vi "Get Required Driver Type.vi"(8 "error in (no error)":errorcluster, 11 "Multi Instrument Msg in":refnum<class "Multi Instrument Msg.lvclass">) -> (0 "error out":errorcluster, 2 "Required Driver Type":refnum<class "Instrument Driver.lvclass">, 3 "Multi Instrument Msg out":refnum<class "Multi Instrument Msg.lvclass">)   [LabVIEW 2020, in "Instrument Handler.lvlib" / "Multi Instrument Msg.lvclass"]
doc: "Get the Required Driver Type for execution of the Instrument Msg.\n\nThis implementation does nothing."
uses:
  Multi Instrument Msg.lvclass
  PPL/HDH.Actor Framework.Core.Instrument Driver.lvlibp/Instrument Driver/Instrument Driver.lvclass
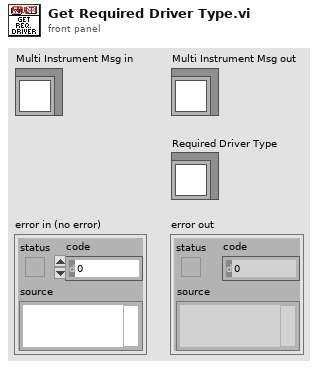
[diagram p1: front panel]
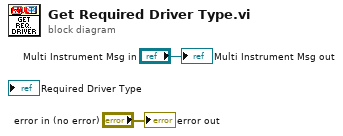
[diagram p0: block diagram]
diagram:
  "error out" <- "error in (no error)"
  "Multi Instrument Msg out" <- "Multi Instrument Msg in"
